vi "Gaussian-Stimulation.vi"(4 "Strength (V)":dbl=10.0, 6 "Delay (ms)":dbl=40.0, 7 "# Samples in":T1 format="%#_9f", 8 "Delay end (ms)":dbl=80.0, 9 "Width of pulse (ms)":dbl=50.0, 11 "Sampling Rate":T1 format="%#_9f") -> (0 "Number of Samples (Total)":dbl, 1 "Array":dbl[](array[numeric]), 2 "Array 2":T1[](array[typedef]) format="%#_9f", 3 "# Samples out":T1 format="%#_9f", 5 "LSCI CCD":cluster{i32, dbl, dbl[]}(graph)={0, 1e-05, array[16000 elements]})   [LabVIEW 2021]
uses:
  Settings.ctl
  <vilib>/Analysis/1siggen.llb/Ramp Pattern by Samples.vi
  <vilib>/Analysis/NI_AALBase.lvlib
panel:
  out "x-y":T1 format="%#_9f"
  out "size(s)":i32
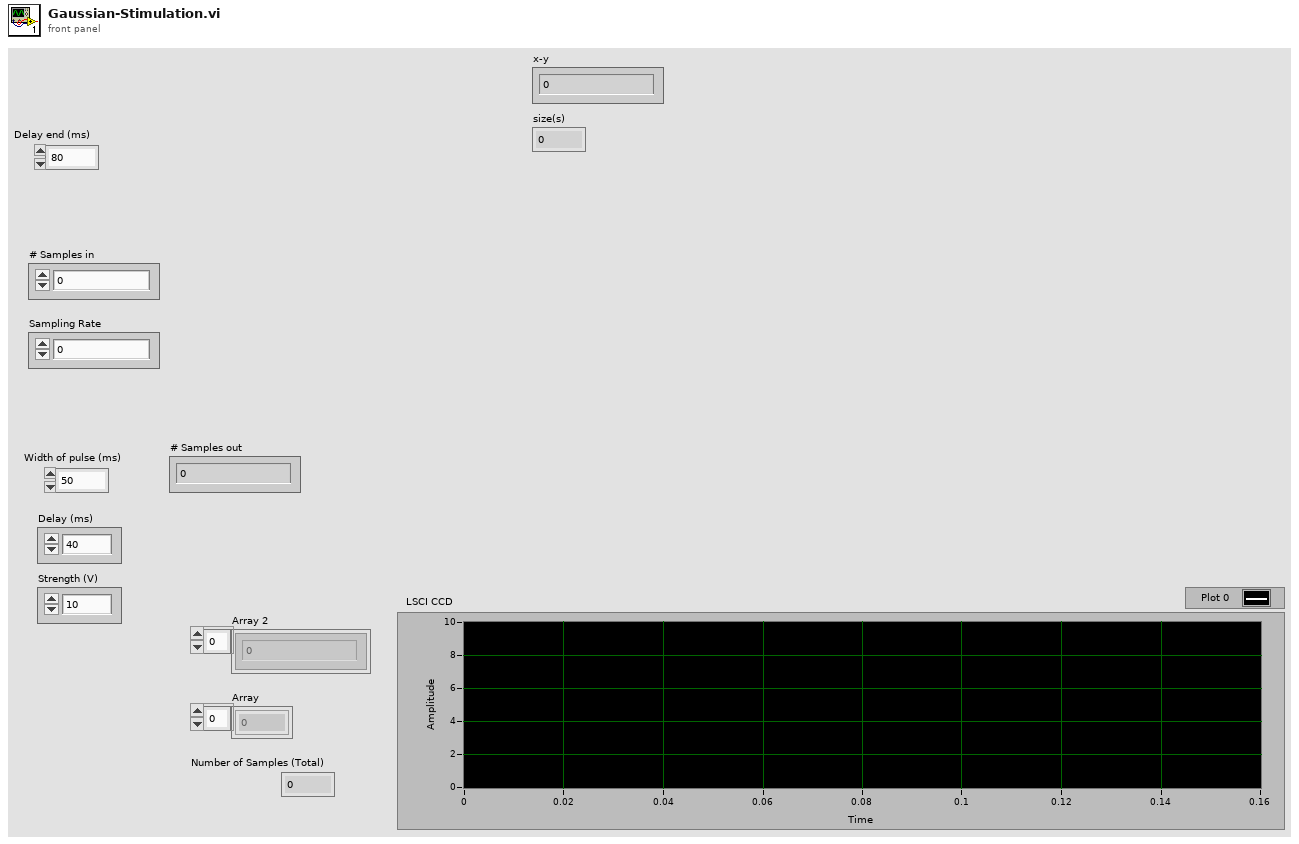
[diagram p1: front panel]
types:
  T1 = typedef "Settings.ctl" = dbl
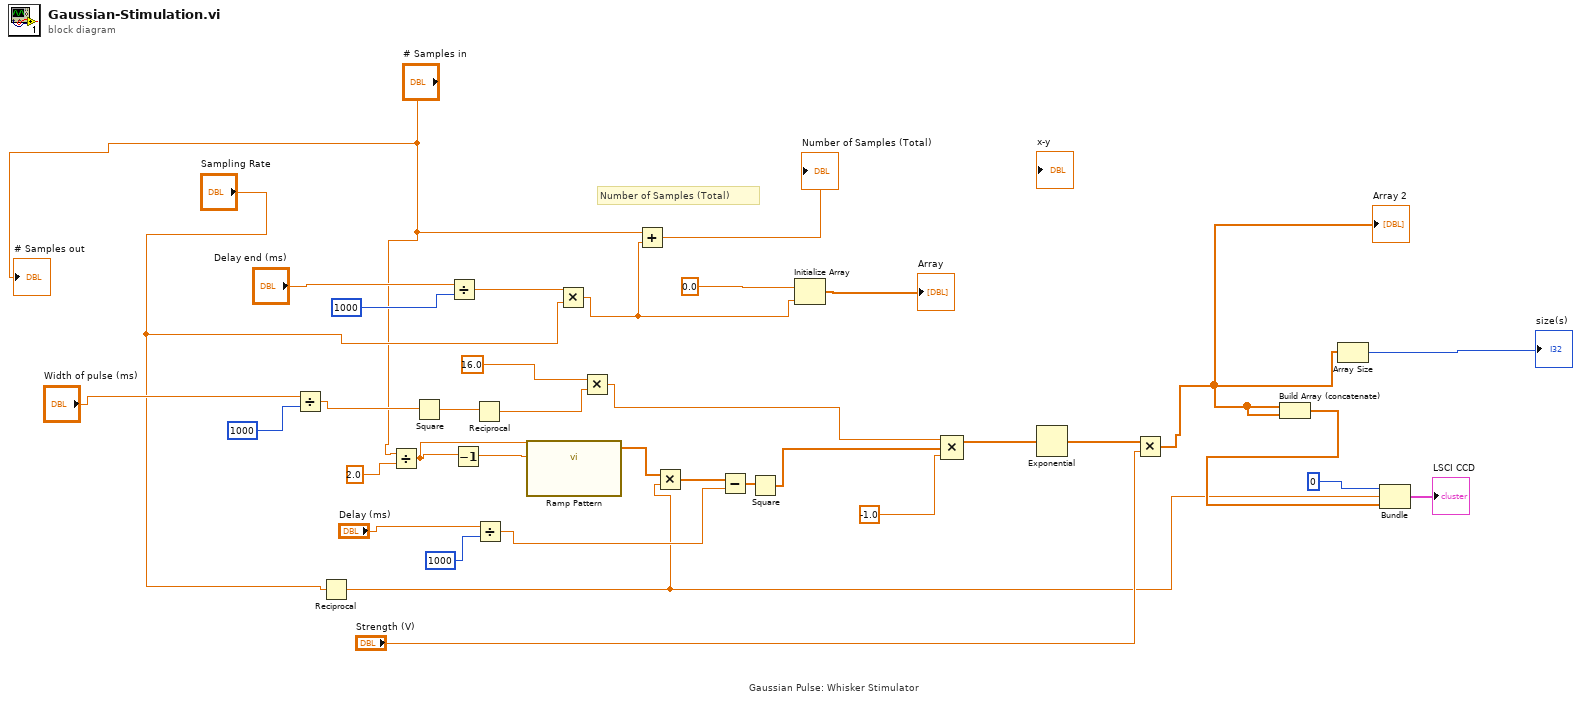
[diagram p0: block diagram]
diagram:
  # "Number of Samples (Total)"
  # "Gaussian Pulse: Whisker Stimulator"
  n1 = Divide(x="Width of pulse (ms)", y=1000) -> (x/y=w32:dbl)
  n2 = Reciprocal(x="Sampling Rate") -> (1/x=w2:T1)
  n3 = Divide(x="# Samples in", y=T1 2.0) -> (x/y=w3:T1)
  n4 = Square(x=w32) -> (x^2=w28:dbl)
  n5 = Divide(x="Delay end (ms)", y=1000) -> (x/y=w35:dbl)
  n6 = Decrement(x=w3) -> (x-1=w20:T1)
  n7 = Reciprocal(x=w28) -> (1/x=w29:dbl)
  n8 = Divide(x="Delay (ms)", y=1000) -> (x/y=w14:dbl)
  n9 = call-poly <vilib>:"Ramp Pattern.vi"("end"=w20, "samples"=w3) -> ("Ramp Pattern"=w21:dbl[])  [unwired: 8 in, 1 out]
  n10 = Multiply(x=w35, y="Sampling Rate") -> (x*y=w36:T1)
  n11 = Multiply(x=16.0, y=w29) -> (x*y=w13:dbl)
  n12 = Add(x="# Samples in", y=w36) -> (x+y=→"Number of Samples (Total)":T1)
  n13 = Multiply(x=w21, y=w2) -> (x*y=w11:T1[])
  n14 = Subtract(x=w11, y=w14) -> (x-y=w22:T1[])
  n15 = Square(x=w22) -> (x^2=w23:T1[])
  n16 = Initialize Array(0.0 ("element"), w36) -> (→"Array":dbl[])
  n17 = Compound Arithmetic op=MULTIPLY(w13, w23, -1.0) -> (w24:T1[])
  n18 = Exponential(1:w24) -> (0:w25:T1[])
  n19 = Multiply(x=w25, y="Strength (V)") -> (x*y=w1:T1[])
  "Array 2" <- w1
  n20 = Build Array (concatenate)(w1, w1) -> (w8:T1[])
  n21 = Array Size(array=w1) -> (size(s)=→"size(s)":i32)
  n22 = Bundle(0, w2, w8) -> (→"LSCI CCD":cluster{i32, T1, T1[]})  [unwired: 1 in]
  "# Samples out" <- "# Samples in"
